vi "setupTestLog.vi"(8 "error in (no error)":errorcluster, 10 "Model in":refnum<class "Model.lvclass">, 11 "Bootloader in":refnum<class "Bootloader.lvclass">) -> (0 "error out":errorcluster, 2 "Model out":refnum<class "Model.lvclass">, 3 "Bootloader out":refnum<class "Bootloader.lvclass">)   [LabVIEW 2015, in "Bootloader.lvclass"]
uses:
  Bootloader.lvclass
  Model/Model.lvclass
  Typedefs/TestLogTypes.ctl
  Model/Model.lvclass/Model.ctl
  TestLogFactory/ITestLogFactory/ITestLogFactory.lvclass
  Typedefs/FAMTTypedefs.lvlib
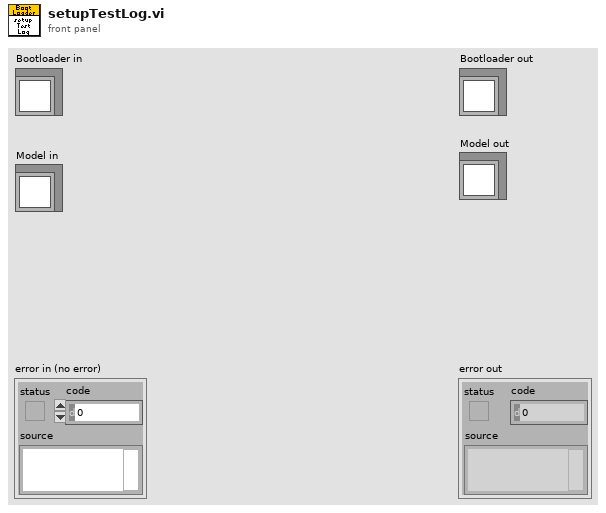
[diagram p1: front panel]
types:
  T1 = typedef "FAMTTypedefs.lvlib/TestLogTypes.ctl" = enum16{"CSV Test Log"}
  T2 = typedef "FAMTTypedefs.lvlib/Scan Settings.ctl" = cluster{"Amplitude Scan Settings":T3, "Rate Scan Settings":T4[], "Sample Count":u32, "Iterations":dbl, "Amplitude":dbl[unit], "Offset":dbl[unit], "Frequency":dbl[unit], "Waveform":T5, "F1":dbl[unit], "F2":dbl[unit], "Duty Cycle":dbl, "ILC Rate":dbl[unit], "Operator":string, "Scan Name":string, "Notes":string}
  T3 = typedef "FAMTTypedefs.lvlib/Test Values.ctl" = cluster{"Start Value":dbl, "Stop Value":dbl, "Steps":u16}
  T4 = typedef "ILCCommon.lvlib/ILCConfiguration.lvlib/Scan Rates.ctl" = enum16{"50", "60", "100", "120", "200", "240", "300", "400", "480", "600", "1200", "2400", "4800"}
  T5 = typedef "FAMTTypedefs.lvlib/Waveform.ctl" = enum16{"Sine Wave", "Triangle Wave", "Square Wave", "Sawtooth Wave", "Chirp Wave", "Gaussian Wave"}
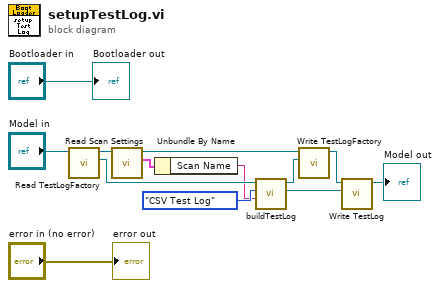
[diagram p0: block diagram]
diagram:
  n1 = call "Read TestLogFactory.vi"("Model in"="Model in") -> ("ITestLogFactory.lvclass"=w11:refnum<class "ITestLogFactory.lvclass">, "Model out"=w2:refnum<class "Model.lvclass">)  [unwired: 9 in]
  n2 = call "Read Scan Settings.vi"("Model in"=w2) -> ("Scan Settings"=w4:T2, "Model out"=w1:refnum<class "Model.lvclass">)  [unwired: 9 in]
  n3 = Unbundle By Name(w4) -> ("Scan Name"=w3:string)
  n4 = call-dynamic "buildTestLog.vi"("Serial Number"=w3, "TestLogTypes"=TestLogTypes."CSV Test Log", "ITestLogFactory in"=w11) -> ("ITestLog"=w9:refnum<class "ITestLog.lvclass">, "ITestLogFactory out"=w10:refnum<class "ITestLogFactory.lvclass">)  [unwired: 6 in, 1 out]
  n5 = call "Write TestLogFactory.vi"("ITestLogFactory.lvclass"=w10, "Model in"=w1) -> ("Model out"=w8:refnum<class "Model.lvclass">)  [unwired: 9 in]
  n6 = call "Write TestLog.vi"("ITestLog.lvclass"=w9, "Model in"=w8) -> ("Model out"=→"Model out":refnum<class "Model.lvclass">)  [unwired: 9 in]
  "error out" <- "error in (no error)"
  "Bootloader out" <- "Bootloader in"
